vi "XYStage.ReadPosition(counts).vi"(8 "error in (no error)":errorcluster, 11 "XYStage":refnum<class "XYStage.lvclass">) -> (0 "error out":errorcluster, 2 "Counts":T1, 3 "XYStage out":refnum<class "XYStage.lvclass">)   [LabVIEW 2013, in "XYStage.lvclass"]
doc: "---------------------------------------------------------------\nJKI State Machine Objects™\nhttp://jki.net/state-machine-objects/\nCopyright (C) 2005-2015, JKI <info@jki.net>\nALL RIGHTS RESERVEDJKI State Machine Objects (SMO) 1.0.0.5\nJKI - JKI\nCopyright (c) 2016, JKI"
uses:
  XYStage.lvclass
  Typedefs/(counts)Coords--Cluster.ctl
panel:
  # "For instructions on how to use the JKI State Machine Objects, examples and video tutorials, visit:\nhttp://jki.net/state-machine-objects/\n\nJKI State Machine Objects™\nhttp://jki.net/state-machine-objects/\nCopyright (C) 2005-2015, JKI <info@jki.net>\nALL RIGHTS RESERVED"
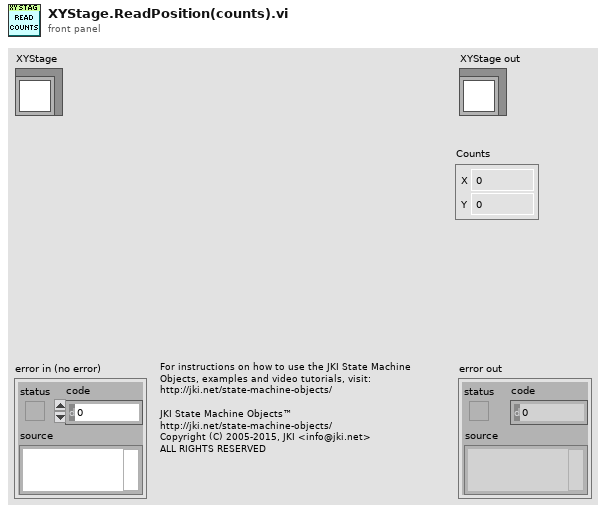
[diagram p1: front panel]
types:
  T1 = typedef "XYStage.lvclass/(counts)Coords--Cluster.ctl" = cluster{"X":i32, "Y":i32}
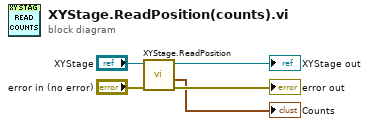
[diagram p0: block diagram]
diagram:
  n1 = call-dynamic "XYStage.ReadPosition.vi"("error in (no error)"="error in (no error)", "XYStage"="XYStage") -> ("error out"=→"error out":errorcluster, "Counts out"=→"Counts":T1, "XYStage out"=→"XYStage out":refnum<class "XYStage.lvclass">)  [unwired: 6 in, 1 out]
